vi "GT Clear Event.vi"(8 "error in (no error)":errorcluster caption="错误输入（无错误）", 11 "cardNum":i16) -> (0 "error out":errorcluster caption="错误输出", 3 "cardNum":i16)   [LabVIEW 2020, in "gts1.lvlib"]
doc: "GT_API GT_ClearEvent(short cardNum);"
uses:
  gts1.lvlib
  dll/32bit/multi_card/gts.dll
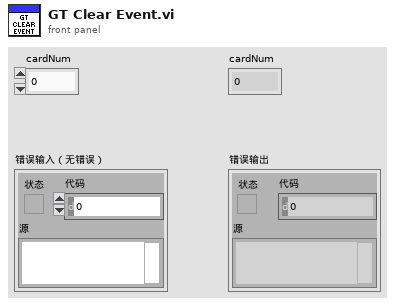
[diagram p1: front panel]
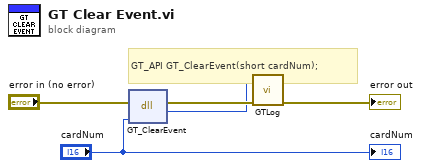
[diagram p0: block diagram]
diagram:
  # "GT_API GT_ClearEvent(short cardNum);"
  n1 = dll-call lib="D:/Git/GoogolCard/dll/32bit/multi_card/gts.dll" fn="GT_ClearEvent"(error in="error in (no error)", "cardNum"="cardNum") -> (error out=w4:errorcluster, w2:i16)  [unwired: 3 in, 1 out]
  n2 = call "GTLog.vi"("error in (no error)"=w4, "Numeric"=w2) -> ("error out"=→"error out":errorcluster)  [unwired: 9 in]
  "cardNum" <- "cardNum"
